vi "layout.vi"(0 "reference":refnum<class "Graph.lvclass">, 1 "LayoutNodes(Empty=All)":refnum<class "AbstractNode.lvclass">[](array[class]), 5 "error in (no error)":errorcluster) -> (14 "reference out":refnum<class "Graph.lvclass">, 19 "error out":errorcluster)   [LabVIEW 2016, in "Graph.lvclass"]
doc: "public void layout()"
uses:
  <resource>/Framework/Providers/Open_GDS/UML/Graph_class/Graph.lvclass
  <resource>/Framework/Providers/Open_GDS/UML/AbstractNode_class/AbstractNode.lvclass
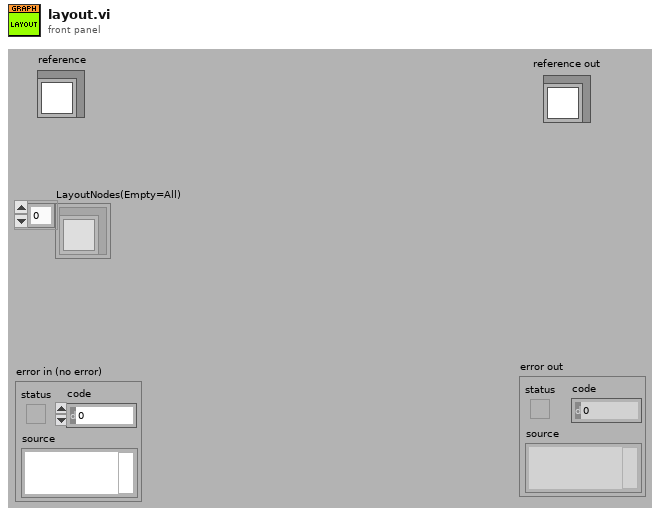
[diagram p1: front panel]
types:
  T1 = typedef "Graph.lvclass/ObjectAttributes.ctl" = cluster{"nodes":refnum<class "AbstractNode.lvclass">[], "edges":refnum<class "AbstractEdge.lvclass">[], "nodesToBeRemoved":refnum<class "AbstractNode.lvclass">[], "edgesToBeRemoved":refnum<class "AbstractEdge.lvclass">[], "needsLayout":bool, "LayoutNodes":refnum<class "AbstractNode.lvclass">[]}
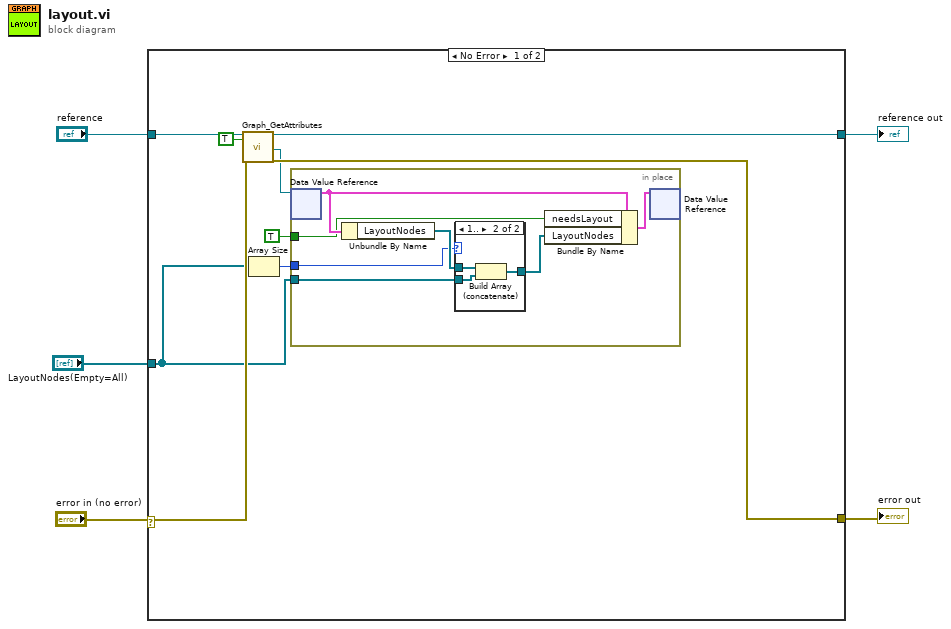
[diagram p0: block diagram]
diagram:
  n1 = case shown="No Error" "error in (no error)" {
    selector: "error in (no error)" -> [w11 w25]
    tunnel: "reference" -> [w14 w26]
    tunnel: [w13 w25] -> w4
    tunnel: [w12 w26] -> w3
    tunnel: "LayoutNodes(Empty=All)" -> [w6 _]
    frame No Error {
      n2 = call <resource>:"Graph_GetAttributes.vi"("reference in"=w14, "OnlyGetDvrReference(False)"=TRUE, "error in (no error)"=w11) -> ("reference out"=w12:refnum<class "Graph.lvclass">, "DataRef"=w9:refnum<data-value>, "error out"=w13:errorcluster)  [unwired: 13 in, 1 out]
      n3 = Array Size(array=w6) -> (size(s)=w7:i32)
      n4 = in-place {
        in-place-border: TRUE ("needsLayout") -> [w19]
        in-place-border: w7 -> [w16]
        in-place-border: w6 -> [w15]
        n5 = in-place-dvr #1(w9) -> (w21:T1)  [unwired: 1 out]
        n6 = Unbundle By Name(w21) -> ("LayoutNodes"=w20:refnum<class "AbstractNode.lvclass">[])
        n7 = case shown="1.." w16 {
          tunnel: w20 -> [_ w24]
          tunnel: [_ w23] -> w18
          tunnel: w15 -> [_ w22]
          frame 0, Default {
          }
          frame 1.. {
            n8 = Build Array (concatenate)(w24, w22) -> (w23:refnum<class "AbstractNode.lvclass">[])
          }
        }
        n9 = Bundle By Name(cluster=w21, "needsLayout"=w19, "LayoutNodes"=w18) -> (w17:T1)
        n10 = in-place-dvr #1(w17) -> ()  [unwired: 2 out]
      }
    }
    frame Error {
    }
  }
  "reference out" <- w3
  "error out" <- w4
